vi "AO add remove elements.vi"(1 "NewVal in":T1 {"AO f (Hz)" min=0.001 max=10000.0; "AO DC (V)" format="%.3p"; "AO Amp (V)" format="%.3p"}) -> (0 "NewVal out":T1 {"AO f (Hz)" min=0.001 max=10000.0; "AO DC (V)" format="%.3p"; "AO Amp (V)" format="%.3p"})   [LabVIEW 2016, in "Instrument.Lockin.lvclass"]
uses:
  Instrument.Lockin.lvclass
  LockinDAQ/Typedefs/AO-cluster.ctl
  LockinDAQ/Typedefs/AO_Amp-array.ctl
  LockinDAQ/Typedefs/AO_DC-array.ctl
  LockinDAQ/Typedefs/AO_f-array.ctl
  LockinDAQ/Typedefs/AO_phi-array.ctl
  LockinDAQ/Typedefs/Function-array.ctl
  LockinDAQ/Typedefs/Function-enum.ctl
  LockinDAQ/LockinDAQ.lvclass
panel:
  # "1"
  # "2"
  # "3"
  # "4"
  # "5"
  # "6"
  # "7"
  # "8"
  # "1"
  # "2"
  # "3"
  # "4"
  # "5"
  # "6"
  # "7"
  # "8"
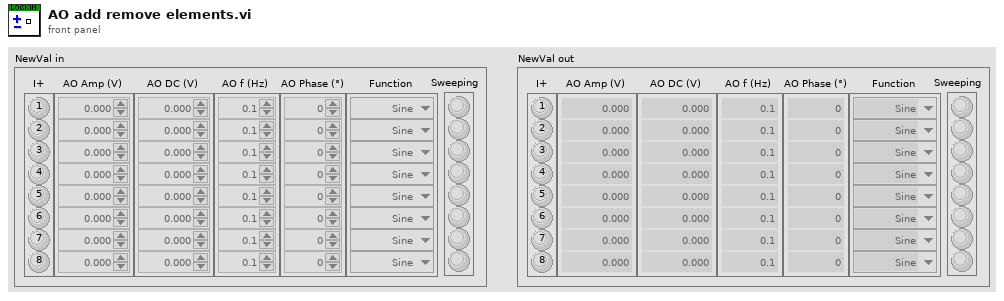
[diagram p1: front panel]
types:
  T1 = typedef "LockinDAQ.lvclass/AO-cluster.ctl" = cluster{"AO Amp (V)":T2, "AO DC (V)":T3, "AO f (Hz)":T4, "AO Phase (°)":T5, "Function":T6, "I+":bool[], "Sweeping":bool[]}
  T2 = typedef "LockinDAQ.lvclass/AO_Amp-array.ctl" = dbl[]
  T3 = typedef "LockinDAQ.lvclass/AO_DC-array.ctl" = dbl[]
  T4 = typedef "LockinDAQ.lvclass/AO_f-array.ctl" = dbl[]
  T5 = typedef "LockinDAQ.lvclass/AO_phi-array.ctl" = dbl[]
  T6 = typedef "LockinDAQ.lvclass/Function-array.ctl" = T7[]
  T7 = typedef "LockinDAQ.lvclass/Function-enum.ctl" = enum16{"Sine", "Triangle", "Square", "Sawtooth"}
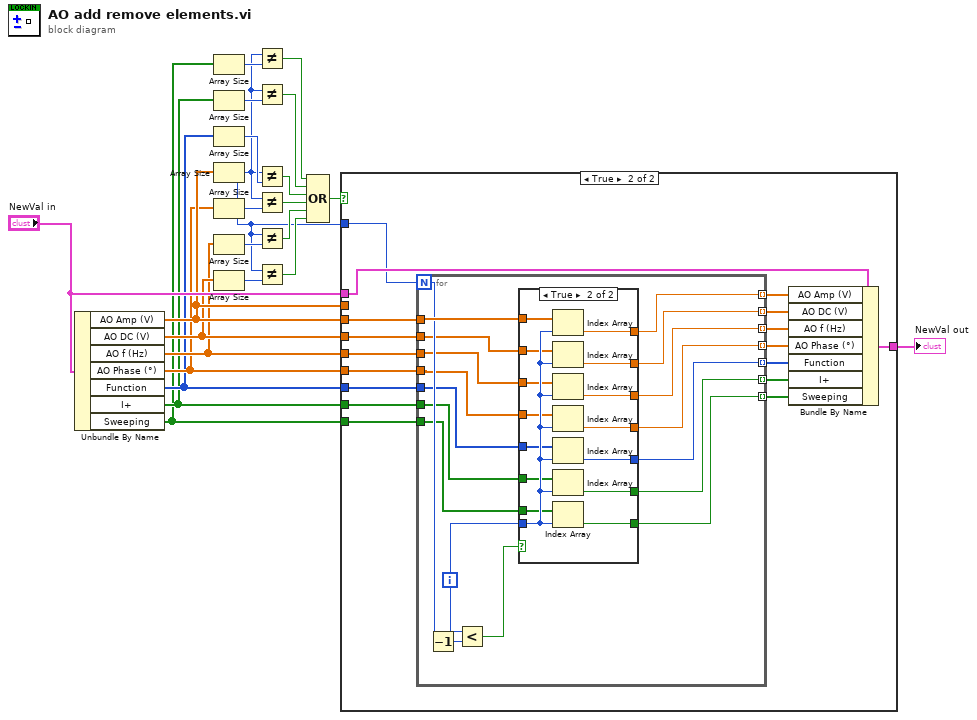
[diagram p0: block diagram]
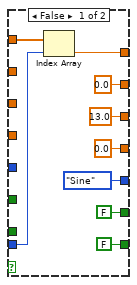
[diagram p3: hidden frame]
diagram:
  n1 = Unbundle By Name("NewVal in") -> ("AO Amp (V)"=w7:T2, "AO DC (V)"=w6:T3, "AO f (Hz)"=w5:T4, "AO Phase (°)"=w4:T5, "Function"=w3:T6, "I+"=w2:bool[], "Sweeping"=w1:bool[])
  n2 = Array Size(array=w1) -> (size(s)=w16:i32)
  n3 = Array Size(array=w2) -> (size(s)=w17:i32)
  n4 = Array Size(array=w3) -> (size(s)=w18:i32)
  n5 = Array Size(array=w7) -> (size(s)=w8:i32)
  n6 = Array Size(array=w4) -> (size(s)=w19:i32)
  n7 = Array Size(array=w5) -> (size(s)=w20:i32)
  n8 = Array Size(array=w6) -> (size(s)=w21:i32)
  n9 = Not Equal?(x=w8, y=w16) -> (x != y?=w15:bool)
  n10 = Not Equal?(x=w8, y=w17) -> (x != y?=w14:bool)
  n11 = Not Equal?(x=w8, y=w18) -> (x != y?=w13:bool)
  n12 = Not Equal?(x=w8, y=w19) -> (x != y?=w12:bool)
  n13 = Not Equal?(x=w8, y=w20) -> (x != y?=w11:bool)
  n14 = Not Equal?(x=w8, y=w21) -> (x != y?=w10:bool)
  n15 = Compound Arithmetic op=OR(w15, w14, w13, w12, w11, w10) -> (w9:bool)
  n16 = case shown="True" w9 {
    tunnel: [w24 w41] -> w23
    tunnel: "NewVal in" -> [w24 w40]
    tunnel: w7 -> [_ _]
    tunnel: w8 -> [_ w36]
    tunnel: w7 -> [_ w35]
    tunnel: w6 -> [_ w34]
    tunnel: w5 -> [_ w33]
    tunnel: w4 -> [_ w32]
    tunnel: w3 -> [_ w31]
    tunnel: w2 -> [_ w30]
    tunnel: w1 -> [_ w29]
    frame False {
    }
    frame True {
      n17 = for {
        N: w36 -> [w57]
        tunnel: [w52] -> w26 mode=indexing
        tunnel: [w56] -> w39 mode=indexing
        tunnel: [w55] -> w38 mode=indexing
        tunnel: [w51] -> w28 mode=indexing
        tunnel: [w50] -> w37 mode=indexing
        tunnel: w35 -> [w59]
        tunnel: w34 -> [w44]
        tunnel: w33 -> [w45]
        tunnel: w32 -> [w47]
        tunnel: w31 -> [w46]
        tunnel: w30 -> [w48]
        tunnel: w29 -> [w49]
        tunnel: [w54] -> w27 mode=indexing
        tunnel: [w53] -> w25 mode=indexing
        i -> [w58]
        n18 = Decrement(x=w57) -> (x-1=w42:i32)
        n19 = Less?(x=w58, y=w42) -> (x < y?=w43:bool)
        n20 = case shown="True" w43 {
          tunnel: w59 -> [w68 w83]
          tunnel: w58 -> [w67 w82]
          tunnel: [w66 w69] -> w56
          tunnel: [0.0 ("AO DC") w81] -> w55
          tunnel: [13.0 ("AO f") w80] -> w54
          tunnel: [0.0 ("AO phi") w79] -> w53
          tunnel: [Function-enum."Sine" ("Signal Type") w78] -> w52
          tunnel: [FALSE ("Boolean") w77] -> w51
          tunnel: [FALSE ("Boolean") w76] -> w50
          tunnel: w49 -> [_ w75]
          tunnel: w48 -> [_ w74]
          tunnel: w47 -> [_ w73]
          tunnel: w46 -> [_ w72]
          tunnel: w45 -> [_ w71]
          tunnel: w44 -> [_ w70]
          frame False {
            n21 = Index Array(array=w68, index=w67) -> (element=w66:dbl)
          }
          frame True {
            n22 = Index Array(array=w83, index=w82) -> (element=w69:dbl)
            n23 = Index Array(array=w70, index=w82) -> (element=w81:dbl)
            n24 = Index Array(array=w71, index=w82) -> (element=w80:dbl)
            n25 = Index Array(array=w73, index=w82) -> (element=w79:dbl)
            n26 = Index Array(array=w72, index=w82) -> (element=w78:T7)
            n27 = Index Array(array=w74, index=w82) -> (element=w77:bool)
            n28 = Index Array(array=w75, index=w82) -> (element=w76:bool)
          }
        }
      }
      n29 = Bundle By Name(cluster=w40, "AO Amp (V)"=w39, "AO DC (V)"=w38, "AO f (Hz)"=w27, "AO Phase (°)"=w25, "Function"=w26, "I+"=w28, "Sweeping"=w37) -> (w41:T1)
    }
  }
  "NewVal out" <- w23
